vi "initialize.vi"(8 "error in (no error)":errorcluster, 11 "ColorOverlay in":refnum<class "ColorOverlay.lvclass">) -> (0 "error out":errorcluster, 3 "ColorOverlay out":refnum<class "ColorOverlay.lvclass">)   [LabVIEW 2010, in "ColorOverlay.lvclass"]
uses:
  ColorOverlay.lvclass
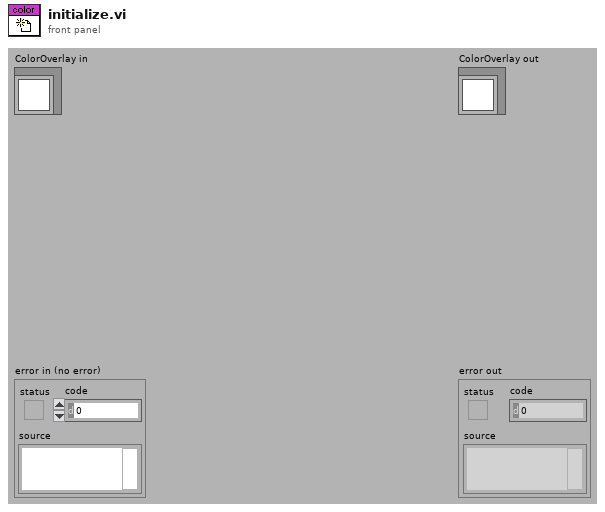
[diagram p1: front panel]
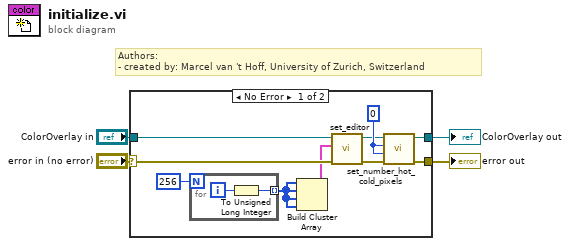
[diagram p0: block diagram]
diagram:
  # "Authors: \n- created by: Marcel van 't Hoff, University of Zurich, Switzerland"
  n1 = case shown="No Error" "error in (no error)" {
    selector: "error in (no error)" -> [w9 w18]
    tunnel: [w8 w18] -> w3
    tunnel: [w10 w17] -> w1
    tunnel: "ColorOverlay in" -> [w11 w17]
    frame No Error {
      w14 = 0 ("# cold pixels")
      n2 = for {
        N: 256 -> [_]
        tunnel: [w15] -> w7 mode=indexing
        i -> [w16]
        n3 = To Unsigned Long Integer(number=w16) -> (unsigned 32bit integer=w15:u32)
      }
      n4 = Build Cluster Array(w7, w7, w7, w7) -> (w5:cluster{u32[]}[])
      n5 = call-dynamic "set_editor.vi"("error in (no error)"=w9, "graph editor"=w5, "ColorOverlay in"=w11) -> ("error out"=w12:errorcluster, "ColorOverlay out"=w13:refnum<class "ColorOverlay.lvclass">)  [unwired: 7 in]
      n6 = call-dynamic "set_number_hot_cold_pixels.vi"("error in (no error)"=w12, "# hot pixels"=w14, "# cold pixels"=w14, "ColorOverlay in"=w13) -> ("error out"=w8:errorcluster, "ColorOverlay out"=w10:refnum<class "ColorOverlay.lvclass">)  [unwired: 6 in]
    }
    frame Error {
    }
  }
  "error out" <- w3
  "ColorOverlay out" <- w1
